vi "Write Channel List.vi"(8 "error in (no error)":errorcluster, 10 "Channel List":i8[](array[numeric]), 11 "Generic Data Acquisition in":refnum<class "Generic Data Acquisition.lvclass">) -> (0 "error out":errorcluster, 3 "Generic Data Acquisition out":refnum<class "Generic Data Acquisition.lvclass">)   [LabVIEW 2016, in "Generic Data Acquisition.lvlib" / "Generic Data Acquisition.lvclass"]
uses:
  Generic Data Acquisition.lvclass
  Generic Data Acquisition.lvclass/Generic Data Acquisition.ctl
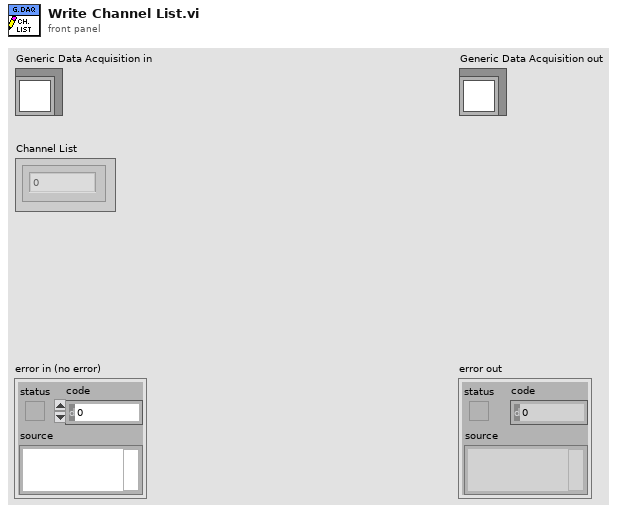
[diagram p1: front panel]
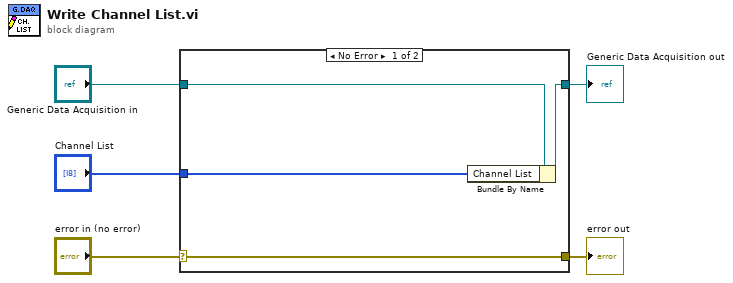
[diagram p0: block diagram]
diagram:
  n1 = case shown="No Error" "error in (no error)" {
    selector: "error in (no error)" -> [w9 w10]
    tunnel: [w9 w10] -> w4
    tunnel: [w7 w11] -> w2
    tunnel: "Generic Data Acquisition in" -> [w8 w11]
    tunnel: "Channel List" -> [w6 _]
    frame No Error {
      n2 = Bundle By Name(cluster=w8, "Channel List"=w6) -> (w7:refnum<class "Generic Data Acquisition.lvclass">)
    }
    frame Error {
    }
  }
  "error out" <- w4
  "Generic Data Acquisition out" <- w2
